vi "ELVIS III v1.0 RPC Garbage Collection.vi"(8 "error in (no error)":errorcluster) -> (0 "error out":errorcluster)   [LabVIEW 2021]
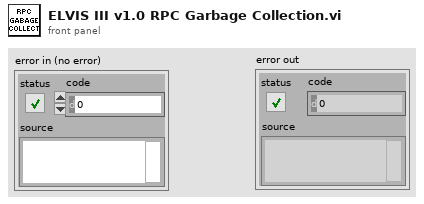
[diagram p1: front panel]
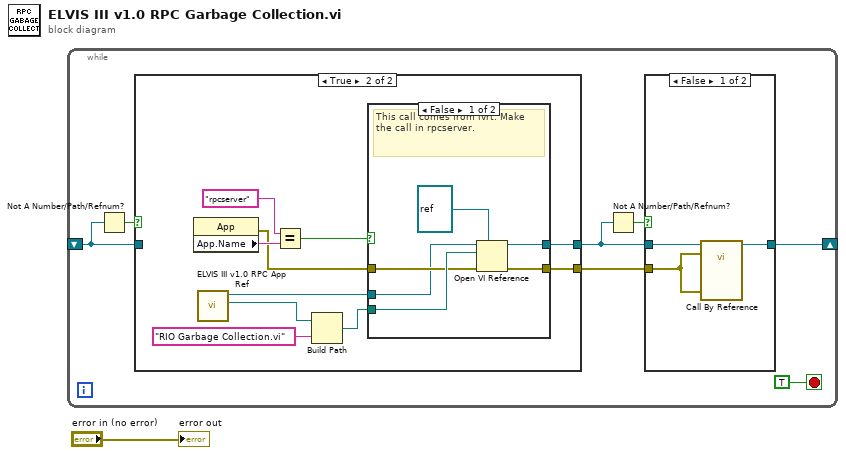
[diagram p0: block diagram]
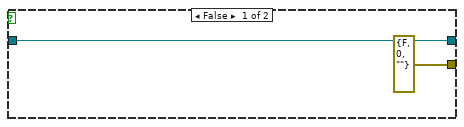
[diagram p2: hidden frame]
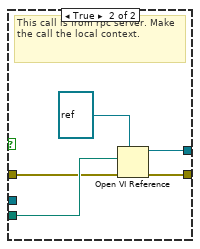
[diagram p3: hidden frame]
diagram:
  n1 = while {
    shift-right: [w5] -> _
    shift-left: _ -> [w3]
    stop <- TRUE stop-if-true
    n2 = Not A Number/Path/Refnum?(number/path/refnum=w3) -> (NaN/Path/Refnum?=w4:bool)
    n3 = case shown="True" w4 {
      tunnel: [w10 w17] -> w7
      tunnel: w3 -> [w10 _]
      tunnel: [errorcluster {"status"=FALSE, "code"=0, "source"=""} ("error out") w15] -> w2
      frame False {
      }
      frame True {
        n4 = property class="App"() -> (error out=w16:errorcluster, "App.Name"=w20:string)  [unwired: 2 in, 1 out]
        n5 = call <vilib>:"ELVIS III v1.0 RPC App Ref.vi"() -> ("Lib Path"=w12:path, "RPC Reference"=w14:refnum<vi>)  [unwired: 10 in]
        n6 = Equal?(x="rpcserver" ("Application:Name"), y=w20) -> (x = y?=w19:bool)
        n7 = Build Path(base path=w12, name or relative path="RIO Garbage Collection.vi") -> (appended path=w11:path)
        n8 = case shown="False" w19 {
          tunnel: [w25 w30] -> w17
          tunnel: w11 -> [w24 w29]
          tunnel: w16 -> [w22 w27]
          tunnel: [w23 w28] -> w15
          tunnel: w14 -> [w21 _]
          frame False {
            # "This call comes from lvrt. Make the call in rpcserver."
            n9 = Open VI Reference(type specifier VI Refnum (for type only)=refnum<vi> refnum, application reference (local)=w21, vi path=w24, error in (no error)=w22) -> (vi reference=w25:refnum<vi>, error out=w23:errorcluster)  [unwired: 2 in]
          }
          frame True {
            # "This call is from rpc server. Make the call the local context."
            n10 = Open VI Reference(type specifier VI Refnum (for type only)=refnum<vi> refnum, vi path=w29, error in (no error)=w27) -> (vi reference=w30:refnum<vi>, error out=w28:errorcluster)  [unwired: 3 in]
          }
        }
      }
    }
    n11 = Not A Number/Path/Refnum?(number/path/refnum=w7) -> (NaN/Path/Refnum?=w8:bool)
    n12 = case shown="False" w8 {
      tunnel: w7 -> [w34 w35]
      tunnel: [w33 w35] -> w5
      tunnel: w2 -> [w32 _]
      frame False {
        n13 = call-by-ref "?"(reference=w34, error in=w32, "error in"=w32) -> (reference out=w33:refnum<vi>)  [unwired: 10 in, 2 out]
      }
      frame True {
        # "The call is not available. The target is installed by 19.0. Ignore for backward compatibility."
      }
    }
  }
  "error out" <- "error in (no error)"
